vi "Zeit.vi"   [LabVIEW 2010]
uses:
  GVAbschalten.vi
  GVZeitZyklus.vi
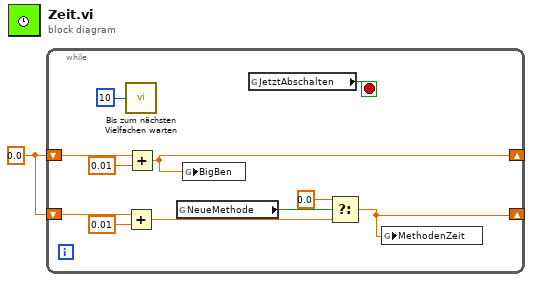
[diagram p0: block diagram]
diagram:
  w1 = 0.0
  n1 = while {
    shift-right: [w8] -> _
    shift-left: w1 -> [w10]
    shift-right: [w2] -> _
    shift-left: w1 -> [w7]
    stop <- w12 stop-if-true
    n2 = call "Bis zum nächsten Vielfachen warten"("Count(mSec)"=u32 10) -> ()  [unwired: 1 out]
    n3 = Add(x=w7, y=0.01) -> (x+y=w5:dbl)
    n4 = Add(x=w10, y=0.01) -> (x+y=w8:dbl)
    n5 = global read "GVAbschalten.vi" "NeueMethode"() -> (w3:bool)
    n6 = global write "GVZeitZyklus.vi" "BigBen"(w8) -> ()
    n7 = global read "GVAbschalten.vi" "JetztAbschalten"() -> (w12:bool)
    n8 = Select(t=0.0, s=w3, f=w5) -> (s? t:f=w2:dbl)
    n9 = global write "GVZeitZyklus.vi" "MethodenZeit"(w2) -> ()
  }
